vi "DAQ Circular Buffer.vi"(8 "# of Samples":i32, 9 "# of Channels":i32, 10 "Mode":enum16{"Initialize", "Read", "Write"}(ring), 11 "Data to Write":sgl[][](array[numeric]) format="%.2f") -> (0 "Max Buffer Size":i32, 1 "Current Buffer Size":i32, 3 "Data Read":sgl[][](array[numeric]) format="%.2f")   [LabVIEW 2019]
doc: "This VI is used in many locations throughout the program as a data buffer. It serves mainly two purposes. In alarms and logging, the DAQ data, whether scaled or voltage, is entered into the buffer. In other parts of the program, data is read from the buffer. Its length is always two minutes regardless of sample rate."
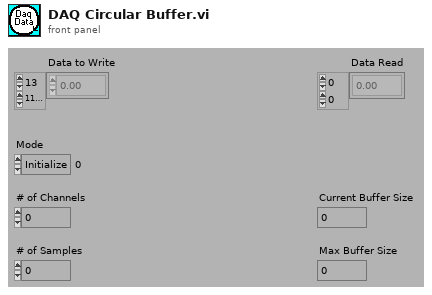
[diagram p1: front panel]
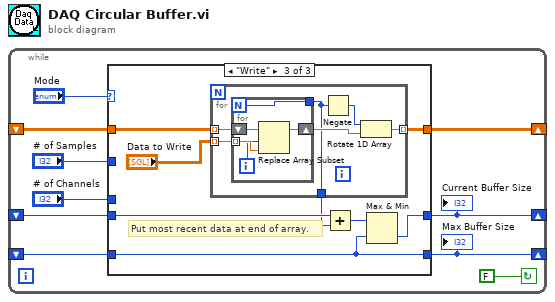
[diagram p0: block diagram]
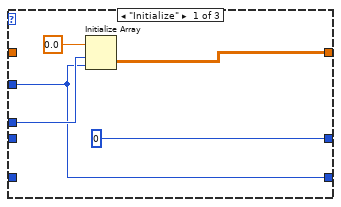
[diagram p2: hidden frame]
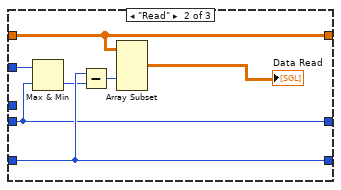
[diagram p3: hidden frame]
diagram:
  n1 = while {
    shift-left: _ -> [w4]
    shift-right: [w2] -> _
    shift-left: _ -> [w5]
    shift-right: [w3] -> _
    shift-left: _ -> [w8]
    shift-right: [w9] -> _
    stop <- FALSE continue-if-true
    n2 = case shown="\"Write\"" "Mode" {
      tunnel: [w14 w22 w28] -> w9
      tunnel: w8 -> [_ w22 w29]
      tunnel: "# of Channels" -> [w12 _ _]
      tunnel: "# of Samples" -> [w11 w19 _]
      tunnel: [0 w18 w23] -> w3
      tunnel: w5 -> [_ w18 w27]
      tunnel: [w11 w20 w24] -> w2
      tunnel: w4 -> [_ w20 w24]
      frame "Initialize" {
        n3 = Initialize Array(sgl 0.0, w12, w11) -> (w14:sgl[][])
      }
      frame "Read" {
        n4 = Max & Min(x=w19, y=w18) -> (min(x,y)=w17:i32)  [unwired: 1 out]
        n5 = Subtract(x=w20, y=w17) -> (x-y=w21:i32)
        n6 = Array Subset(array=w22, index (col)=w21) -> (→"Data Read":sgl[][])  [unwired: 3 in]
      }
      frame "Write" {
        # "Put most recent data at end of array."
        n7 = for {
          tunnel: "Data to Write" -> [w36] mode=indexing
          tunnel: w29 -> [w34] mode=indexing
          tunnel: [w33] -> w28 mode=indexing
          tunnel: [w31] -> w26
          n8 = for {
            N -> [w37]
            shift-right: [w40] -> w35
            shift-left: w34 -> [w41]
            tunnel: w36 -> [w39] mode=indexing
            tunnel: [w37] -> w31
            i -> [w38]
            n9 = Replace Array Subset(array=w41, new element=w39, index=w38) -> (w40:sgl[])
          }
          n10 = Negate(x=w31) -> (-x=w32:i32)
          n11 = Rotate 1D Array(1:w35, 2:w32) -> (0:w33:sgl[])
        }
        n12 = Add(x=w27, y=w26) -> (x+y=w25:i32)
        n13 = Max & Min(x=w25, y=w24) -> (min(x,y)=w23:i32)  [unwired: 1 out]
      }
    }
    "Current Buffer Size" <- w3
    "Max Buffer Size" <- w2
  }
